vi "Close.vi"(8 "error in (no error)":errorcluster, 11 "RRG in":refnum<class "Eltochpribor RRG.lvclass">) -> (0 "error out":errorcluster)   [LabVIEW 2015, in "Eltochpribor RRG.lvclass"]
doc: "Closes connection to device."
uses:
  Eltochpribor RRG.lvclass
  Modbus Client/PL Modbus Client.lvclass
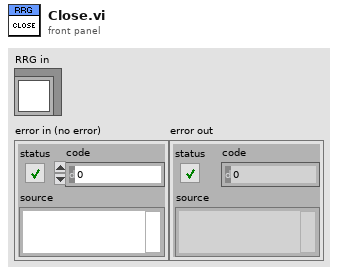
[diagram p1: front panel]
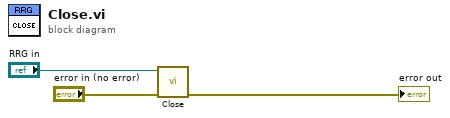
[diagram p0: block diagram]
diagram:
  n1 = call-parent "Close.vi"("error in (no error)"="error in (no error)", "MODBUS in"="RRG in") -> ("error out"=→"error out":errorcluster)  [unwired: 9 in]
